vi "DropletDB-GFV.vi"(8 "error in (no error)":errorcluster, 10 "Data in":variant, 11 "Command In":T1=enum."Init") -> (0 "error out":errorcluster, 2 "Data out":variant)   [LabVIEW 2013]
uses:
  DbEnum.ctl
  TypeDef/GreyLevelData.ctl
  TypeDef/FreezePointData.ctl
  DropletDB.ctl
  ConfEnum.ctl
  ConfDB.ctl
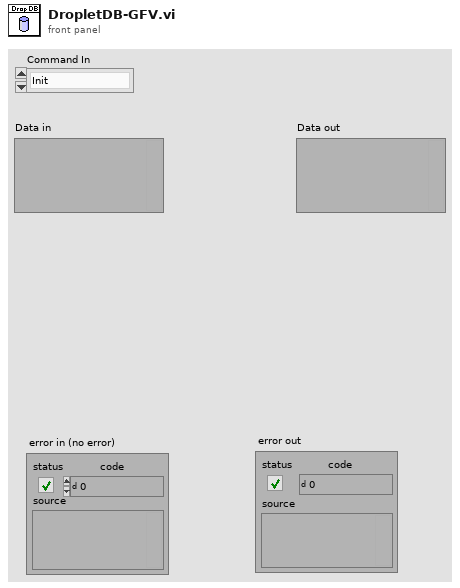
[diagram p1: front panel]
types:
  T1 = typedef "DbEnum.ctl" = enum16{"Write DropletDB", "Init", "Insert Detection Result Data", "Insert Grey Level Result", "Insert Baseline Results", "AddFreezeImagesAtCertainDroplet", "UpdateIncludeDroplet", "Insert Freeze Analysis Results", "GetDropDB", "GetNoFreezedDroplets", "GetGreyLevelAndDiff", "GetGreyLevelatIndexTime", "GetDropletsBoundingBox"}
  T2 = cluster{"Position":cluster{"x":sgl, "y":sgl}, "Angle":sgl, "Scale":sgl, "Score":sgl, "Bounding Box":cluster{"x":sgl, "y":sgl}[]}[]
  T3 = typedef "DropletDB.ctl" = cluster{"ImageFreezeIndex":i32, "DropIndex":i32, "Position":cluster{"x":sgl, "y":sgl}, "Bounding Box":cluster{"x":sgl, "y":sgl}[], "Score":sgl, "GreyLevelInBoundingBox":dbl[], "GLDifference":dbl[], "Baseline level":dbl, "Peak":cluster{"Value":dbl, "Index":u32}, "Peak Onset":cluster{"Value":dbl, "Index":u32}, "FreezeFileName":string, "FreezeAbsTime":timestamp, "FreezeTemperature":dbl, "ImageIndexArray":u32[], "Freeze Point Found":bool, "Baseline std":dbl, "FreezedImageArray":cluster{"Image":u8[][]}[], "Include Droplet":bool, "Remark":string, "Freeze Rel Time":u32[]}[]
  T4 = typedef "GreyLevelData.ctl" = cluster{"Grey Level":dbl[], "Grey level diff":dbl[], "ImageIndex":u32, "Drop Index":u32}
  T5 = typedef "FreezePointData.ctl" = cluster{"Freeze YesNo":cluster{"Freeze Grey Diff value":dbl, "Freeze Point Found":bool, "Freeze Indices":u32[]}[], "Rel Time":u32[]}
  T6 = cluster{"DropletBaseline":dbl[], "DropletBaselineSTD":dbl[]}
  T7 = typedef "ConfDB.ctl" = cluster{"NumberOfImages":i32, "NoImages2SaveAroundFreeze":i32, "Path":path, "NameOfPartialFile":string, "StartIndex":i32, "NumberOfStdTol":i32, "Detla t (sec)":i32, "Number of images for baseline":i32, "Temperature File Name":string, "Score":dbl, "Index number of Files":i32[], "End Index":i32, "Temperature Array":dbl[], "TStartIndex":i32}
  T8 = typedef "ConfEnum.ctl" = enum16{"Init", "GetConfDB", "GetTemperatureAtIndex", "WriteConfDB", "Configure DB"}
  T9 = cluster{"ImageFreezeIndex":i32, "DropIndex":i32, "Position":cluster{"x":sgl, "y":sgl}, "Bounding Box":cluster{"x":sgl, "y":sgl}[], "Score":sgl, "GreyLevelInBoundingBox":dbl[], "GLDifference":dbl[], "Baseline level":dbl, "Peak":cluster{"Value":dbl, "Index":u32}, "Peak Onset":cluster{"Value":dbl, "Index":u32}, "FreezeFileName":string, "FreezeAbsTime":timestamp, "FreezeTemperature":dbl, "ImageIndexArray":u32[], "Freeze Point Found":bool, "Baseline std":dbl, "FreezedImageArray":cluster{"Image":u8[][]}[], "Include Droplet":bool, "Remark":string, "Freeze Rel Time":u32[]}
  T10 = cluster{"Freeze Grey Diff value":dbl, "Freeze Point Found":bool, "Freeze Indices":u32[]}[]
  T11 = cluster{"ImageFreezeIndex":i32, "DropIndex":i32, "Position":cluster{"x":sgl, "y":sgl}, "Bounding Box":cluster{"x":sgl, "y":sgl}[], "Score":sgl, "GreyLevelInBoundingBox":dbl[], "GLDifference":dbl[], "Baseline level":dbl, "Peak":cluster{"Value":dbl, "Index":u32}, "Peak Onset":cluster{"Value":dbl, "Index":u32}, "FreezeFileName":string, "FreezeAbsTime":timestamp, "FreezeTemperature":dbl, "ImageIndexArray":u32[], "Freeze Point Found":bool, "Baseline std":dbl, "FreezedImageArray":cluster{"Image":u8[][]}[], "Include Droplet":bool, "Remark":string, "Freeze Rel Time":u32[]}[]
  T12 = cluster{"ImageIndexArray":u32[], "GreyLevelInBoundingBox":dbl[][], "GLDifference":dbl[][]}
  T13 = typedef "Image Type" = u32
  T14 = typedef "IMAQ Image.ctl" = refnum<image>
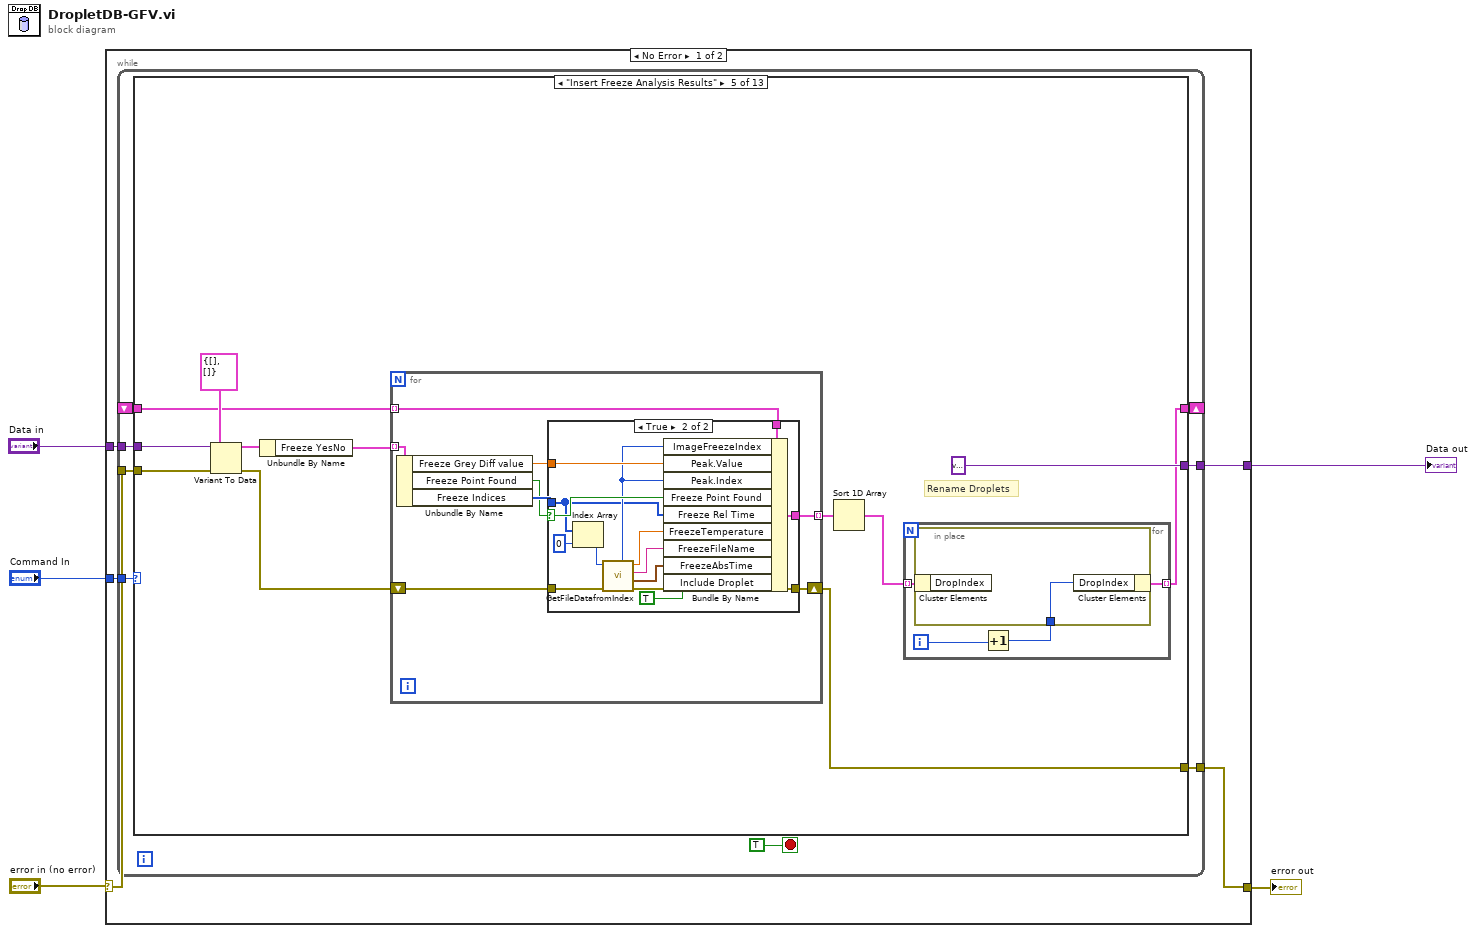
[diagram p0: block diagram]
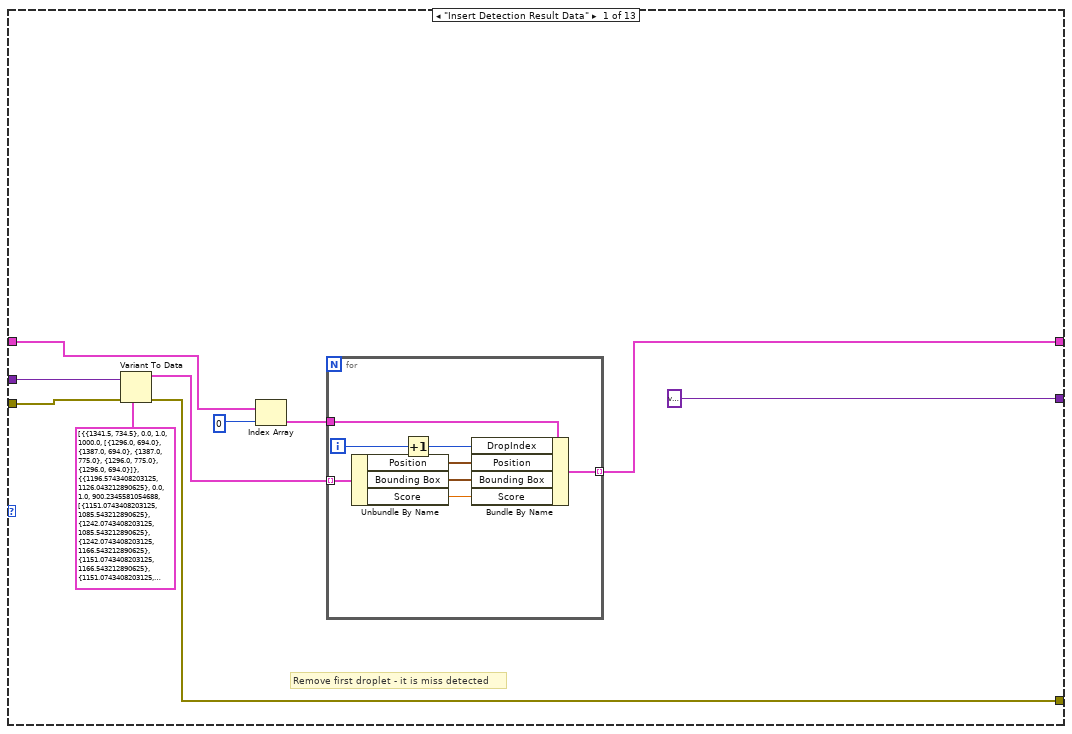
[diagram p2: hidden frame]
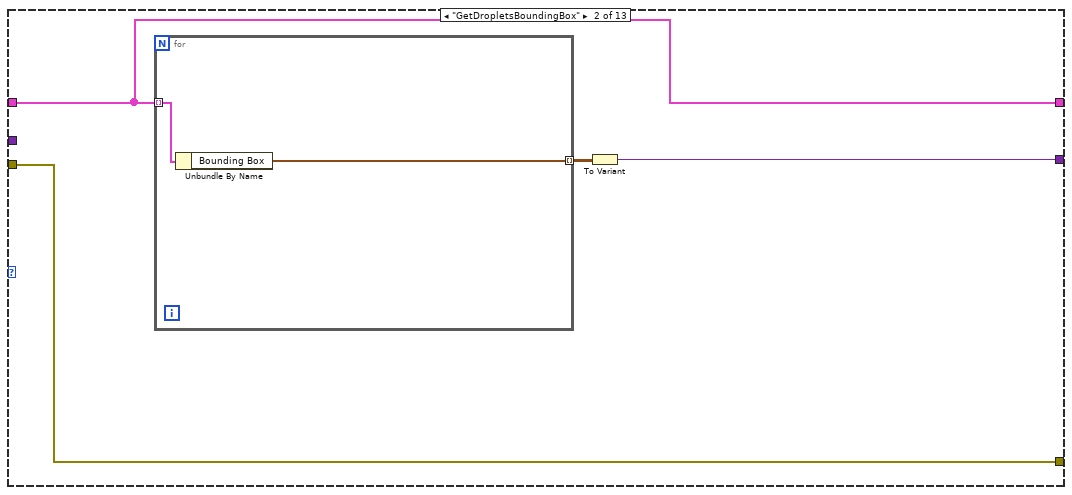
[diagram p3: hidden frame]
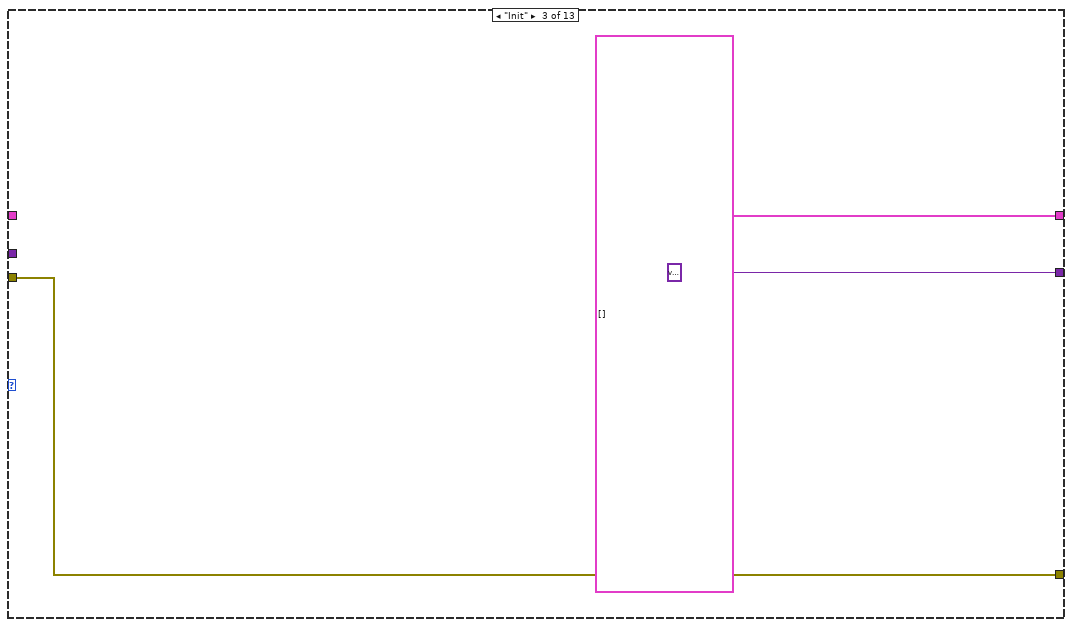
[diagram p4: hidden frame]
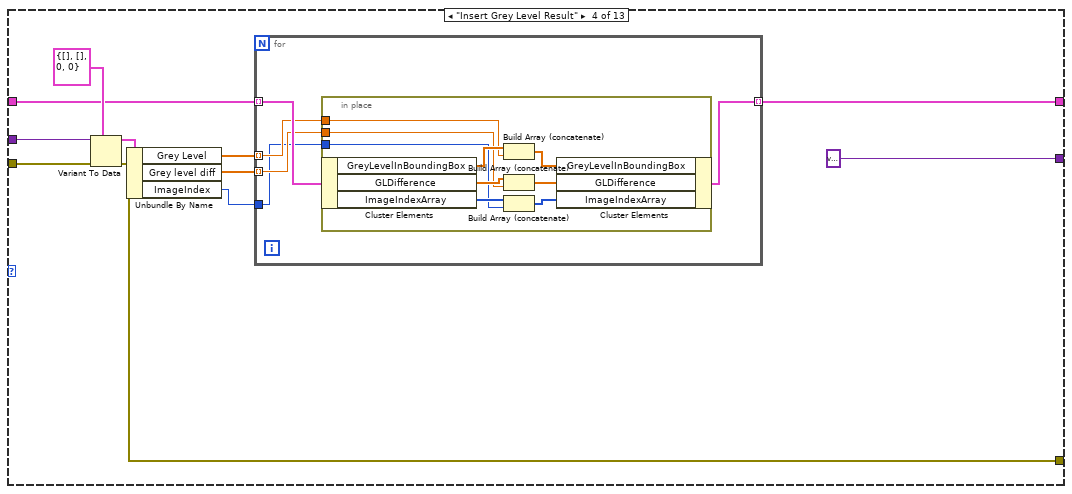
[diagram p5: hidden frame]
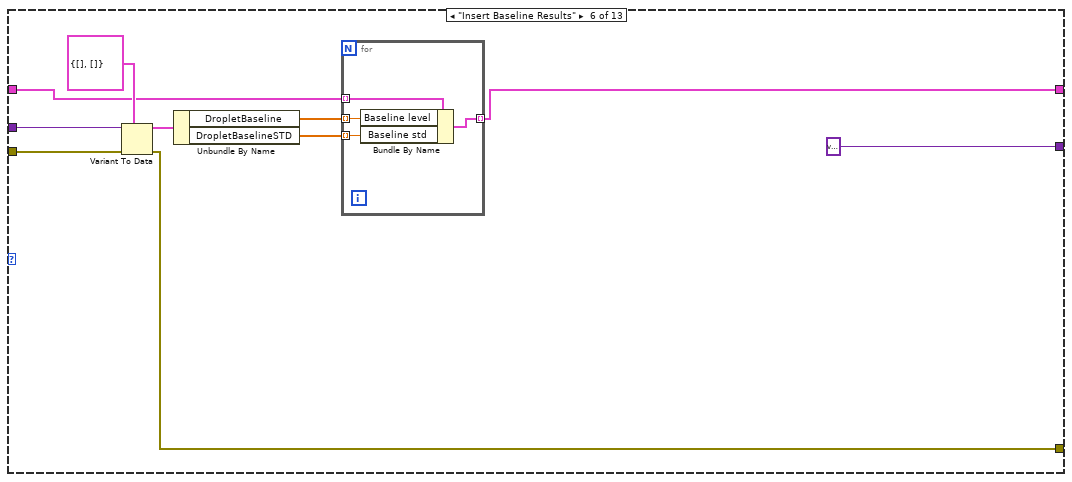
[diagram p7: hidden frame]
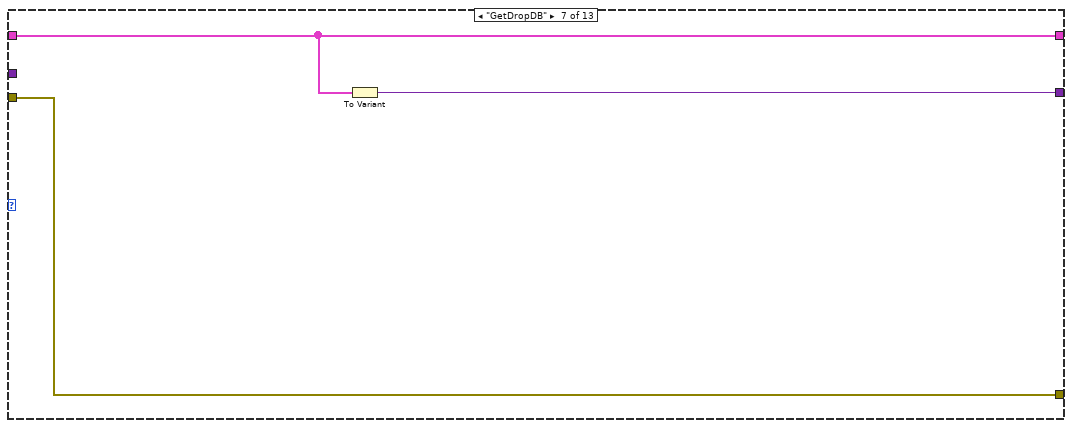
[diagram p8: hidden frame]
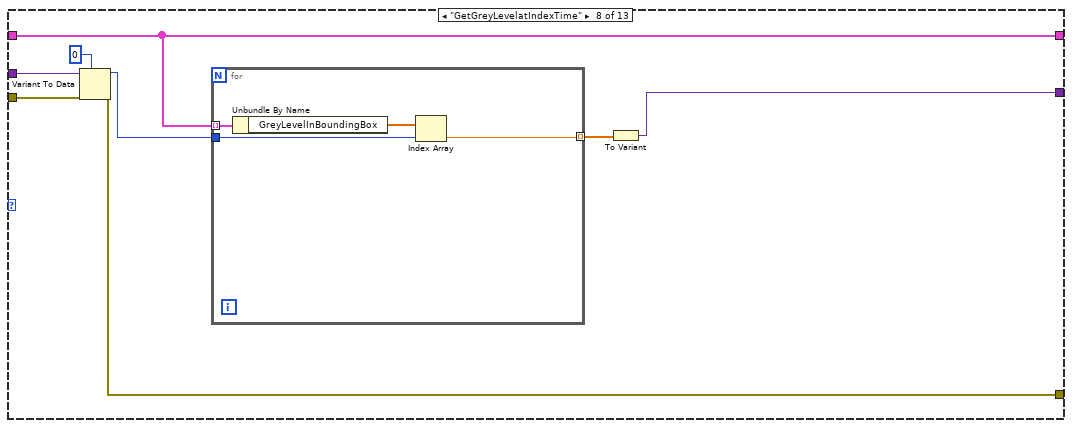
[diagram p9: hidden frame]
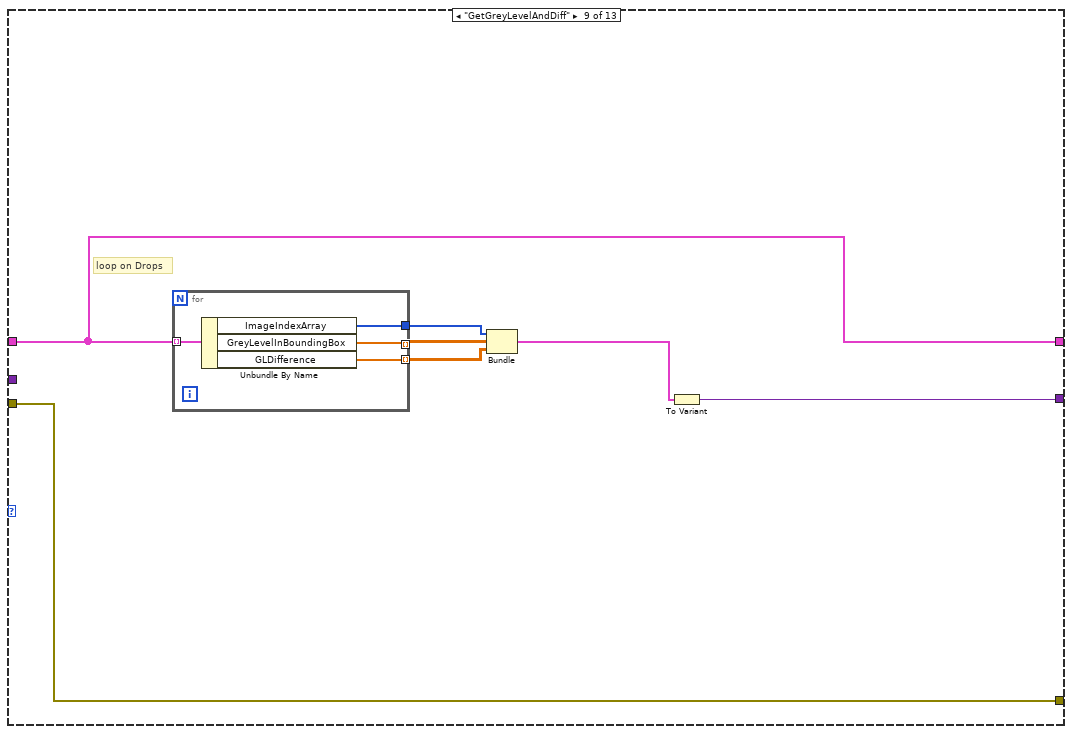
[diagram p10: hidden frame]
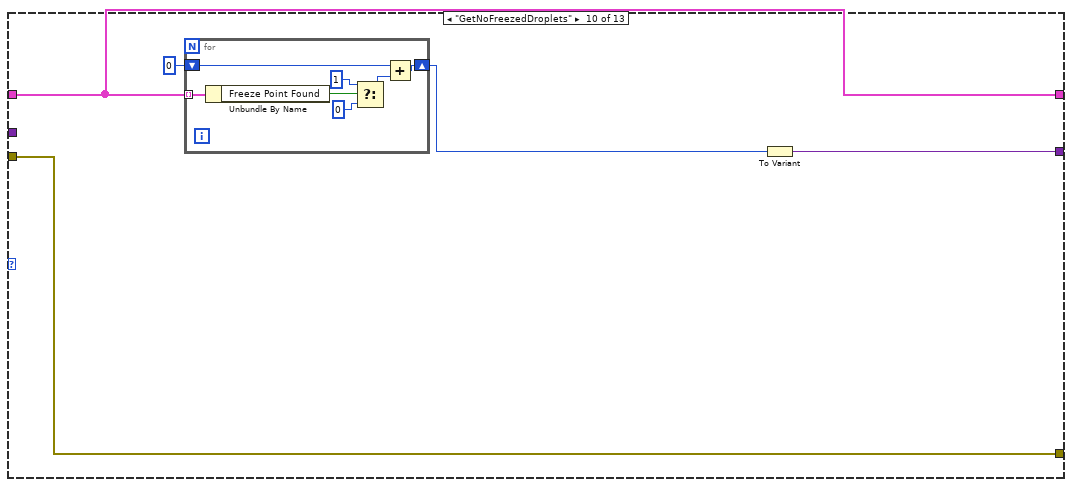
[diagram p11: hidden frame]
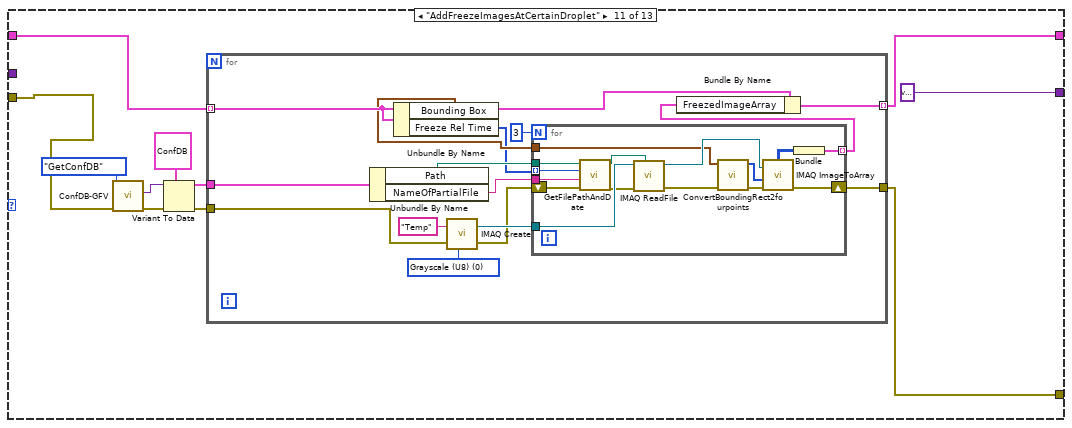
[diagram p12: hidden frame]
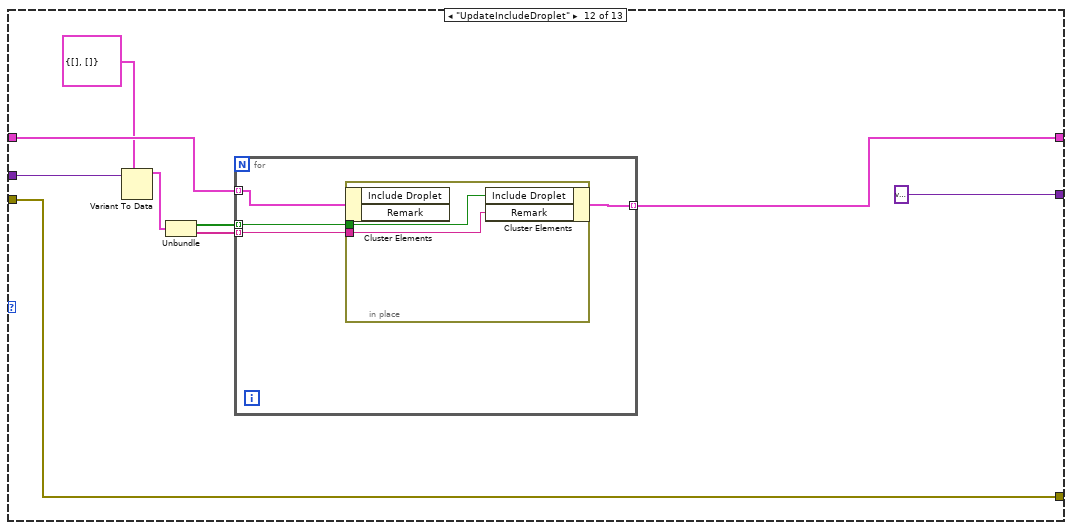
[diagram p13: hidden frame]
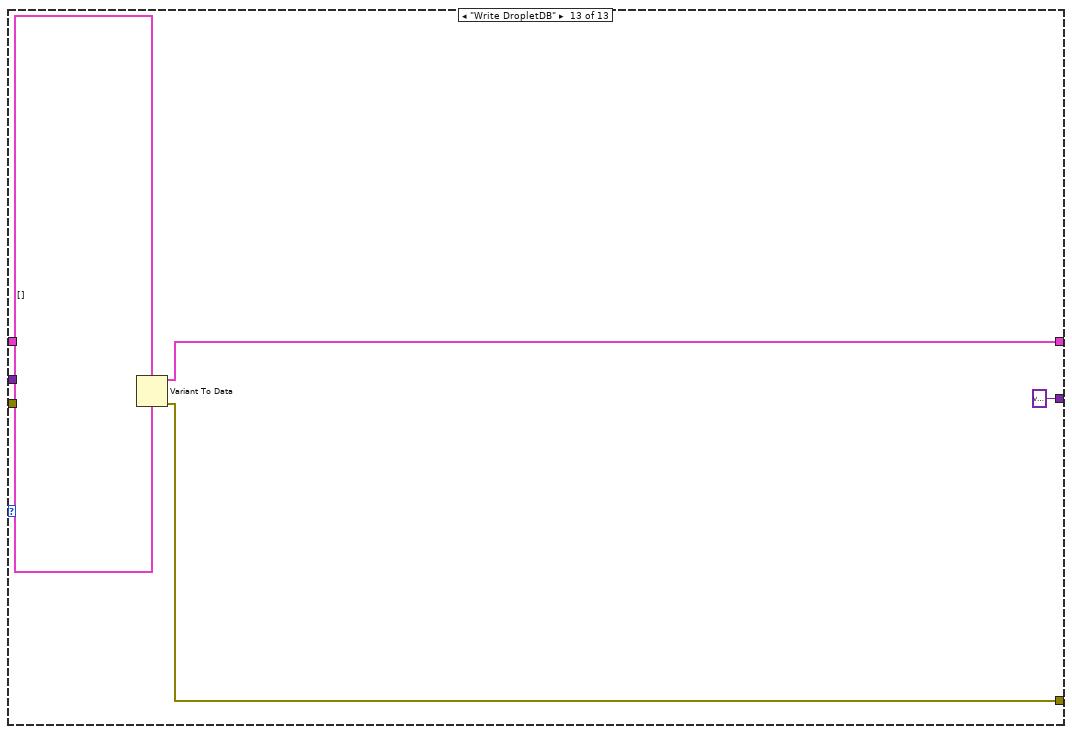
[diagram p14: hidden frame]
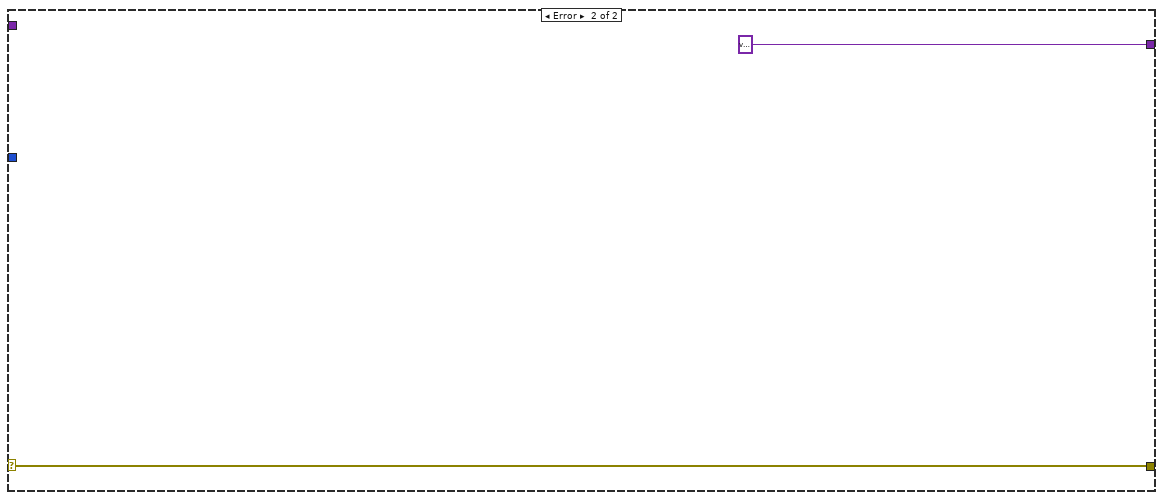
[diagram p15: hidden frame]
diagram:
  n1 = case shown="No Error" "error in (no error)" {
    selector: "error in (no error)" -> [w7 w227]
    tunnel: [w6 w227] -> w4
    tunnel: "Command In" -> [w10 _]
    tunnel: "Data in" -> [w9 _]
    tunnel: [w8 variant ("Variant")] -> w1
    frame No Error {
      n2 = while {
        tunnel: w10 -> [w17]
        shift-right: [w16] -> _
        shift-left: _ -> [w14]
        tunnel: w9 -> [w15]
        tunnel: [w13] -> w8
        tunnel: w7 -> [w12]
        tunnel: [w11] -> w6
        stop <- TRUE stop-if-true
        n3 = case shown="\"Insert Freeze Analysis Results\"" w17 {
          tunnel: [w22 w40 T3 [] ("DropletArray") w47 w72 w114 w128 w134 w147 w155 w166 w209 w222] -> w16
          tunnel: w15 -> [w28 _ _ w56 w82 w120 _ w136 _ _ _ w211 w225]
          tunnel: w14 -> [w23 w40 _ w50 w78 w118 w128 w134 w147 w155 w165 w210 _]
          tunnel: [variant ("Variant") w38 variant ("Variant") variant ("Variant") variant ("Variant") variant ("Variant") w127 w131 w146 w154 variant ("Variant") variant ("Variant") variant ("Variant")] -> w13
          tunnel: w12 -> [w20 w37 w43 w52 w81 w121 w126 w130 w141 w152 w164 w213 w224]
          tunnel: [w19 w37 w43 w51 w75 w112 w126 w129 w141 w152 w167 w213 w221] -> w11
          frame "Insert Detection Result Data" {
            # "Remove first droplet - it is miss detected"
            n4 = Variant To Data(error in=w20, type=T2 [{"Position"={"x"=1341.5, "y"=734.5}, "Angle"=0.0, "Scale"=1.0, "Score"=1000.0, "Bounding Box"=[{"x"=1296.0, "y"=694.0}, {"x"=1387.0, "y"=694.0}, {"x"=1387.0, "y"=775.0}, {"x"=1296.0, "y"=775.0}, {"x"=1296.0, "y"=694.0}]}, {"Position"={"x"=1196.5743, "y"=1126.0432}, "Angle"=0.0, "Scale"=1.0, "Score"=900.23456, "Bounding Box"=[{"x"=1151.0743, "y"=1085.5432}, {"x"=1242.0743, "y"=1085.5432}, {"x"=1242.0743, "y"=1166.5432}, {"x"=1151.0743, "y"=1166.5432}, {"x"=1151.0743, "y"=1085.5432}]}, {"Position"={"x"=1545.7823, "y"=532.04376}, "Angle"=0.0, "Scale"=1.0, "Score"=892.0734, "Bounding Box"=[{"x"=1500.2823, "y"=491.54376}, {"x"=1591.2823, "y"=491.54376}, {"x"=1591.2823, "y"=572.54376}, {"x"=1500.2823, "y"=572.54376}, {"x"=1500.2823, "y"=491.54376}]}, {"Position"={"x"=1094.883, "y"=753.2342}, "Angle"=0.0, "Scale"=1.0, "Score"=891.1741, "Bounding Box"=[{"x"=1049.383, "y"=712.7342}, {"x"=1140.383, "y"=712.7342}, {"x"=1140.383, "y"=793.7342}, {"x"=1049.383, "y"=793.7342}, {"x"=1049.383, "y"=712.7342}]}, {"Position"={"x"=1371.3896, "y"=961.625}, "Angle"=0.0, "Scale"=1.0, "Score"=878.96686, "Bounding Box"=[{"x"=1325.8896, "y"=921.125}, {"x"=1416.8896, "y"=921.125}, {"x"=1416.8896, "y"=1002.125}, {"x"=1325.8896, "y"=1002.125}, {"x"=1325.8896, "y"=921.125}]}, {"Position"={"x"=1686.145, "y"=812.43805}, "Angle"=0.0, "Scale"=1.0, "Score"=825.67773, "Bounding Box"=[{"x"=1640.645, "y"=771.93805}, {"x"=1731.645, "y"=771.93805}, {"x"=1731.645, "y"=852.93805}, {"x"=1640.645, "y"=852.93805}, {"x"=1640.645, "y"=771.93805}]}, {"Position"={"x"=936.9166, "y"=624.4227}, "Angle"=0.0, "Scale"=1.0, "Score"=817.7966, "Bounding Box"=[{"x"=891.4166, "y"=583.9227}, {"x"=982.4166, "y"=583.9227}, {"x"=982.4166, "y"=664.9227}, {"x"=891.4166, "y"=664.9227}, {"x"=891.4166, "y"=583.9227}]}, {"Position"={"x"=1536.802, "y"=1190.3126}, "Angle"=0.0, "Scale"=1.0, "Score"=786.6126, "Bounding Box"=[{"x"=1491.302, "y"=1149.8126}, {"x"=1582.302, "y"=1149.8126}, {"x"=1582.302, "y"=1230.8126}, {"x"=1491.302, "y"=1230.8126}, {"x"=1491.302, "y"=1149.8126}]}, {"Position"={"x"=1679.4249, "y"=1001.6944}, "Angle"=0.0, "Scale"=1.0, "Score"=784.3884, "Bounding Box"=[{"x"=1633.9249, "y"=961.1944}, {"x"=1724.9249, "y"=961.1944}, {"x"=1724.9249, "y"=1042.1943}, {"x"=1633.9249, "y"=1042.1943}, {"x"=1633.9249, "y"=961.1944}]}, {"Position"={"x"=1229.3533, "y"=500.3024}, "Angle"=0.0, "Scale"=1.0, "Score"=773.35645, "Bounding Box"=[{"x"=1183.8533, "y"=459.8024}, {"x"=1274.8533, "y"=459.8024}, {"x"=1274.8533, "y"=540.80237}, {"x"=1183.8533, "y"=540.80237}, {"x"=1183.8533, "y"=459.8024}]}, {"Position"={"x"=951.5936, "y"=1321.2926}, "Angle"=0.0, "Scale"=1.0, "Score"=751.618, "Bounding Box"=[{"x"=906.0936, "y"=1280.7926}, {"x"=997.0936, "y"=1280.7926}, {"x"=997.0936, "y"=1361.7926}, {"x"=906.0936, "y"=1361.7926}, {"x"=906.0936, "y"=1280.7926}]}, {"Position"={"x"=1773.0933, "y"=552.07654}, "Angle"=0.0, "Scale"=1.0, "Score"=723.29376, "Bounding Box"=[{"x"=1727.5933, "y"=511.57654}, {"x"=1818.5933, "y"=511.57654}, {"x"=1818.5933, "y"=592.57654}, {"x"=1727.5933, "y"=592.57654}, {"x"=1727.5933, "y"=511.57654}]}, {"Position"={"x"=1248.5851, "y"=325.4367}, "Angle"=0.0, "Scale"=1.0, "Score"=719.0533, "Bounding Box"=[{"x"=1203.0851, "y"=284.9367}, {"x"=1294.0851, "y"=284.9367}, {"x"=1294.0851, "y"=365.9367}, {"x"=1203.0851, "y"=365.9367}, {"x"=1203.0851, "y"=284.9367}]}, {"Position"={"x"=1253.8042, "y"=1431.3312}, "Angle"=0.0, "Scale"=1.0, "Score"=717.0521, "Bounding Box"=[{"x"=1208.3042, "y"=1390.8312}, {"x"=1299.3042, "y"=1390.8312}, {"x"=1299.3042, "y"=1471.8312}, {"x"=1208.3042, "y"=1471.8312}, {"x"=1208.3042, "y"=1390.8312}]}, {"Position"={"x"=1508.0845, "y"=1397.7313}, "Angle"=0.0, "Scale"=1.0, "Score"=702.3233, "Bounding Box"=[{"x"=1462.5845, "y"=1357.2313}, {"x"=1553.5845, "y"=1357.2313}, {"x"=1553.5845, "y"=1438.2313}, {"x"=1462.5845, "y"=1438.2313}, {"x"=1462.5845, "y"=1357.2313}]}, {"Position"={"x"=1552.1433, "y"=304.62778}, "Angle"=0.0, "Scale"=1.0, "Score"=694.1083, "Bounding Box"=[{"x"=1506.6433, "y"=264.12778}, {"x"=1597.6433, "y"=264.12778}, {"x"=1597.6433, "y"=345.12778}, {"x"=1506.6433, "y"=345.12778}, {"x"=1506.6433, "y"=264.12778}]}, {"Position"={"x"=786.0882, "y"=1109.9098}, "Angle"=0.0, "Scale"=1.0, "Score"=691.0762, "Bounding Box"=[{"x"=740.5882, "y"=1069.4098}, {"x"=831.5882, "y"=1069.4098}, {"x"=831.5882, "y"=1150.4098}, {"x"=740.5882, "y"=1150.4098}, {"x"=740.5882, "y"=1069.4098}]}, {"Position"={"x"=1926.0133, "y"=864.04224}, "Angle"=0.0, "Scale"=1.0, "Score"=639.03375, "Bounding Box"=[{"x"=1880.5133, "y"=823.54224}, {"x"=1971.5133, "y"=823.54224}, {"x"=1971.5133, "y"=904.54224}, {"x"=1880.5133, "y"=904.54224}, {"x"=1880.5133, "y"=823.54224}]}, {"Position"={"x"=1927.5698, "y"=665.46716}, "Angle"=0.0, "Scale"=1.0, "Score"=624.3622, "Bounding Box"=[{"x"=1882.0698, "y"=624.96716}, {"x"=1973.0698, "y"=624.96716}, {"x"=1973.0698, "y"=705.96716}, {"x"=1882.0698, "y"=705.96716}, {"x"=1882.0698, "y"=624.96716}]}, {"Position"={"x"=1036.6719, "y"=924.2498}, "Angle"=0.0, "Scale"=1.0, "Score"=622.71356, "Bounding Box"=[{"x"=991.1719, "y"=883.7498}, {"x"=1082.1719, "y"=883.7498}, {"x"=1082.1719, "y"=964.7498}, {"x"=991.1719, "y"=964.7498}, {"x"=991.1719, "y"=883.7498}]}, {"Position"={"x"=1798.4291, "y"=427.18503}, "Angle"=0.0, "Scale"=1.0, "Score"=612.04645, "Bounding Box"=[{"x"=1752.9291, "y"=386.68503}, {"x"=1843.9291, "y"=386.68503}, {"x"=1843.9291, "y"=467.68503}, {"x"=1752.9291, "y"=467.68503}, {"x"=1752.9291, "y"=386.68503}]}, {"Position"={"x"=679.48035, "y"=781.2287}, "Angle"=0.0, "Scale"=1.0, "Score"=604.38666, "Bounding Box"=[{"x"=633.98035, "y"=740.7287}, {"x"=724.98035, "y"=740.7287}, {"x"=724.98035, "y"=821.7287}, {"x"=633.98035, "y"=821.7287}, {"x"=633.98035, "y"=740.7287}]}, {"Position"={"x"=1858.5896, "y"=1175.5317}, "Angle"=0.0, "Scale"=1.0, "Score"=601.6367, "Bounding Box"=[{"x"=1813.0896, "y"=1135.0317}, {"x"=1904.0896, "y"=1135.0317}, {"x"=1904.0896, "y"=1216.0317}, {"x"=1813.0896, "y"=1216.0317}, {"x"=1813.0896, "y"=1135.0317}]}, {"Position"={"x"=873.6445, "y"=427.1809}, "Angle"=0.0, "Scale"=1.0, "Score"=584.28125, "Bounding Box"=[{"x"=828.1445, "y"=386.6809}, {"x"=919.1445, "y"=386.6809}, {"x"=919.1445, "y"=467.6809}, {"x"=828.1445, "y"=467.6809}, {"x"=828.1445, "y"=386.6809}]}, {"Position"={"x"=599.6848, "y"=551.81195}, "Angle"=0.0, "Scale"=1.0, "Score"=543.92706, "Bounding Box"=[{"x"=554.1848, "y"=511.31195}, {"x"=645.1848, "y"=511.31195}, {"x"=645.1848, "y"=592.31195}, {"x"=554.1848, "y"=592.31195}, {"x"=554.1848, "y"=511.31195}]}] ("Matches (pixel)"), Variant=w28) -> (data=w24:T2, error out=w19:errorcluster)
            n5 = Index Array(array=w23, index=0) -> (element=w25:T9)
            n6 = for {
              tunnel: w24 -> [w31] mode=indexing
              tunnel: [w33] -> w22 mode=indexing
              tunnel: w25 -> [w32]
              i -> [w30]
              n7 = Unbundle By Name(w31) -> ("Position"=w36:cluster{"x":sgl, "y":sgl}, "Bounding Box"=w35:cluster{"x":sgl, "y":sgl}[], "Score"=w34:sgl)
              n8 = Increment(x=w30) -> (x+1=w29:i32)
              n9 = Bundle By Name(cluster=w32, "DropIndex"=w29, "Position"=w36, "Bounding Box"=w35, "Score"=w34) -> (w33:T9)
            }
          }
          frame "GetDropletsBoundingBox" {
            n10 = for {
              tunnel: w40 -> [w42] mode=indexing
              tunnel: [w41] -> w39 mode=indexing
              n11 = Unbundle By Name(w42) -> ("Bounding Box"=w41:cluster{"x":sgl, "y":sgl}[])
            }
            n12 = To Variant(anything=w39) -> (Variant=w38:variant)
          }
          frame "Init" {
          }
          frame "Insert Grey Level Result" {
            n13 = Variant To Data(error in=w52, type=T4 {"Grey Level"=[], "Grey level diff"=[], "ImageIndex"=0, "Drop Index"=0} ("Cluster"), Variant=w56) -> (data=w54:T4, error out=w51:errorcluster)
            n14 = Unbundle By Name(w54) -> ("Grey Level"=w49:dbl[], "Grey level diff"=w48:dbl[], "ImageIndex"=w46:u32)
            n15 = for {
              tunnel: w50 -> [w61] mode=indexing
              tunnel: w49 -> [w60] mode=indexing
              tunnel: w48 -> [w59] mode=indexing
              tunnel: [w58] -> w47 mode=indexing
              tunnel: w46 -> [w57]
              n16 = in-place {
                in-place-border: w60 -> [w68]
                in-place-border: w59 -> [w65]
                in-place-border: w57 -> [w62]
                n17 = in-place-cluster #1(w61) -> ("GreyLevelInBoundingBox"=w70:dbl[], "GLDifference"=w67:dbl[], "ImageIndexArray"=w64:u32[])
                n18 = Build Array (concatenate)(w70, w68) -> (w69:dbl[])
                n19 = Build Array (concatenate)(w67, w65) -> (w66:dbl[])
                n20 = Build Array (concatenate)(w64, w62) -> (w63:u32[])
                n21 = in-place-cluster #1("GreyLevelInBoundingBox"=w69, "GLDifference"=w66, "ImageIndexArray"=w63) -> (w58:T9)
              }
            }
          }
          frame "Insert Freeze Analysis Results" {
            # "Rename Droplets"
            n22 = Variant To Data(error in=w81, type=T5 {"Freeze YesNo"=[], "Rel Time"=[]} ("Freeze YesNo"), Variant=w82) -> (data=w77:T5, error out=w71:errorcluster)
            n23 = Unbundle By Name(w77) -> ("Freeze YesNo"=w76:T10)
            n24 = for {
              tunnel: w76 -> [w95] mode=indexing
              tunnel: w78 -> [w94] mode=indexing
              tunnel: [w92] -> w74 mode=indexing
              shift-right: [w90] -> w75
              shift-left: w71 -> [w91]
              n25 = Unbundle By Name(w95) -> ("Freeze Grey Diff value"=w93:dbl, "Freeze Point Found"=w88:bool, "Freeze Indices"=w89:u32[])
              n26 = case shown="True" w88 {
                selector: w88 -> [_ w103]
                tunnel: w94 -> [w97 w111]
                tunnel: w93 -> [_ w110]
                tunnel: [w97 w109] -> w92
                tunnel: w91 -> [w96 w108]
                tunnel: [w96 w107] -> w90
                tunnel: w89 -> [_ w100]
                frame False {
                }
                frame True {
                  n27 = Index Array(array=w100, index=0) -> (element=w98:u32)
                  n28 = call "GetFileDatafromIndex.vi"("Error In"=w108, "DuplicateFilteredIndex"=w98) -> ("Error Out"=w107:errorcluster, "FreezeAbsTime"=w104:timestamp, "FreezeFileName"=w105:string, "FreezeTemperature"=w106:dbl, "Peak index"=w102:u32)  [unwired: 5 in]
                  n29 = Bundle By Name(cluster=w111, "ImageFreezeIndex"=w102, "Peak.Value"=w110, "Peak.Index"=w102, "Freeze Point Found"=w103, "Freeze Rel Time"=w100, "FreezeTemperature"=w106, "FreezeFileName"=w105, "FreezeAbsTime"=w104, "Include Droplet"=TRUE) -> (w109:T9)
                }
              }
            }
            n30 = Sort 1D Array(array=w74) -> (sorted array=w73:T11)
            n31 = for {
              tunnel: w73 -> [w86] mode=indexing
              tunnel: [w85] -> w72 mode=indexing
              i -> [w84]
              n32 = Increment(x=w84) -> (x+1=w83:i32)
              n33 = in-place {
                in-place-border: w83 -> [w87]
                n34 = in-place-cluster #2(w86) -> ()  [unwired: 1 out]
                n35 = in-place-cluster #2("DropIndex"=w87) -> (w85:T9)
              }
            }
          }
          frame "Insert Baseline Results" {
            n36 = Variant To Data(error in=w121, type=T6 {"DropletBaseline"=[], "DropletBaselineSTD"=[]} ("output cluster"), Variant=w120) -> (data=w117:T6, error out=w112:errorcluster)
            n37 = Unbundle By Name(w117) -> ("DropletBaseline"=w116:dbl[], "DropletBaselineSTD"=w115:dbl[])
            n38 = for {
              tunnel: w118 -> [w125] mode=indexing
              tunnel: w116 -> [w124] mode=indexing
              tunnel: w115 -> [w122] mode=indexing
              tunnel: [w123] -> w114 mode=indexing
              n39 = Bundle By Name(cluster=w125, "Baseline level"=w124, "Baseline std"=w122) -> (w123:T9)
            }
          }
          frame "GetDropDB" {
            n40 = To Variant(anything=w128) -> (Variant=w127:variant)
          }
          frame "GetGreyLevelatIndexTime" {
            n41 = Variant To Data(error in=w130, type=0 ("x-y"), Variant=w136) -> (data=w133:i32, error out=w129:errorcluster)
            n42 = for {
              tunnel: w134 -> [w140] mode=indexing
              tunnel: w133 -> [w138]
              tunnel: [w137] -> w132 mode=indexing
              n43 = Unbundle By Name(w140) -> ("GreyLevelInBoundingBox"=w139:dbl[])
              n44 = Index Array(array=w139, index=w138) -> (element=w137:dbl)
            }
            n45 = To Variant(anything=w132) -> (Variant=w131:variant)
          }
          frame "GetGreyLevelAndDiff" {
            # "loop on Drops"
            n46 = for {
              tunnel: w147 -> [w151] mode=indexing
              tunnel: [w150] -> w144 mode=indexing
              tunnel: [w149] -> w143 mode=indexing
              tunnel: [w148] -> w145
              n47 = Unbundle By Name(w151) -> ("ImageIndexArray"=w148:u32[], "GreyLevelInBoundingBox"=w150:dbl[], "GLDifference"=w149:dbl[])
            }
            n48 = Bundle("ImageIndexArray"=w145, "GreyLevelInBoundingBox"=w144, "GLDifference"=w143) -> (w142:T12)  [unwired: 1 in]
            n49 = To Variant(anything=w142) -> (Variant=w146:variant)
          }
          frame "GetNoFreezedDroplets" {
            n50 = for {
              tunnel: w155 -> [w163] mode=indexing
              shift-right: [w158] -> w153
              shift-left: u32 0 -> [w157]
              n51 = Unbundle By Name(w163) -> ("Freeze Point Found"=w162:bool)
              n52 = Select(t=u32 1, s=w162, f=u32 0) -> (s? t:f=w161:u32)
              n53 = Add(x=w157, y=w161) -> (x+y=w158:u32)
            }
            n54 = To Variant(anything=w153) -> (Variant=w154:variant)
          }
          frame "AddFreezeImagesAtCertainDroplet" {
            n55 = call "ConfDB-GFV.vi"("error in (no error)"=w164, "Command In"=ConfEnum."GetConfDB") -> ("error out"=w171:errorcluster, "Data out"=w172:variant)  [unwired: 8 in]
            n56 = Variant To Data(error in=w171, type=T7 {"NumberOfImages"=0, "NoImages2SaveAroundFreeze"=0, "Path"=path "", "NameOfPartialFile"="", "StartIndex"=0, "NumberOfStdTol"=0, "Detla t (sec)"=0, "Number of images for baseline"=0, "Temperature File Name"="", "Score"=0.0, "Index number of Files"=[], "End Index"=0, "Temperature Array"=[], "TStartIndex"=0} ("ConfDB"), Variant=w172) -> (data=w169:T7, error out=w168:errorcluster)
            n57 = for {
              tunnel: w169 -> [w189]
              tunnel: w168 -> [w188]
              tunnel: [w187] -> w167
              tunnel: w165 -> [w185] mode=indexing
              tunnel: [w186] -> w166 mode=indexing
              w182 = T13 0 items=["Grayscale (U8)", "Grayscale (I16)", "Grayscale (SGL)", "Complex (CSG)", "RGB (U32)", "HSL (U32)", "RGB (U64)", "Grayscale (U16)"] ("Image Type")
              n58 = Unbundle By Name(w189) -> ("Path"=w184:path, "NameOfPartialFile"=w183:string)
              n59 = Unbundle By Name(w185) -> ("Bounding Box"=w176:cluster{"x":sgl, "y":sgl}[], "Freeze Rel Time"=w175:u32[])
              n60 = call "IMAQ Create"("Image Name"="Temp", "Image Type"=w182, "error in (no error)"=w188) -> ("New Image"=w180:T14, "error out"=w179:errorcluster)  [unwired: 1 in, 1 out]
              n61 = for {
                N: 3 -> [_]
                tunnel: w184 -> [w204]
                tunnel: w183 -> [w203]
                tunnel: w180 -> [w201]
                tunnel: [w193] -> w177 mode=indexing
                shift-right: [w192] -> w187
                shift-left: w179 -> [w195]
                tunnel: w176 -> [w191]
                tunnel: w175 -> [w190] mode=indexing
                n62 = call "GetFilePathAndDate.vi"("error in (no error)"=w195, "String"=w203, "Index"=w190, "Path"=w204) -> ("error out"=w196:errorcluster, "file out"=w202:path)  [unwired: 5 in, 1 out]
                n63 = call "IMAQ ReadFile"("File Path"=w202, "error in (no error)"=w196, "Image"=w201) -> ("error out"=w197:errorcluster, "Image Out"=w198:T14)  [unwired: 2 in, 5 out]
                n64 = call "ConvertBoundingRect2fourpoints.vi"("Error In"=w197, "Bounding Box"=w191) -> ("Error Out"=w200:errorcluster, "Array"=w199:i32[])  [unwired: 8 in]
                n65 = call "IMAQ ImageToArray"("error in (no error)"=w200, "Optional Rectangle"=w199, "Image"=w198) -> ("error out"=w192:errorcluster, "Image Pixels (U8)"=w194:u8[][])  [unwired: 1 in, 3 out]
                n66 = Bundle("Image Pixels (U8)"=w194) -> (w193:cluster{"Image Pixels (U8)":u8[][]})  [unwired: 1 in]
              }
              n67 = Bundle By Name(cluster=w185, "FreezedImageArray"=w177) -> (w186:T9)
            }
          }
          frame "UpdateIncludeDroplet" {
            n68 = Variant To Data(type=cluster{bool[], string[]} {[], []} ("cluster"), Variant=w211) -> (data=w207:cluster{bool[], string[]})  [unwired: 1 in, 1 out]
            n69 = Unbundle(w207) -> (w206:bool[], w205:string[])
            n70 = for {
              tunnel: w210 -> [w217] mode=indexing
              tunnel: [w216] -> w209 mode=indexing
              tunnel: w206 -> [w215] mode=indexing
              tunnel: w205 -> [w214] mode=indexing
              n71 = in-place {
                in-place-border: w215 -> [w219]
                in-place-border: w214 -> [w218]
                n72 = in-place-cluster #3(w217) -> ()  [unwired: 2 out]
                n73 = in-place-cluster #3("Include Droplet"=w219, "Remark"=w218) -> (w216:T9)
              }
            }
          }
          frame "Write DropletDB" {
            n74 = Variant To Data(error in=w224, type=T3 [] ("DropletArray"), Variant=w225) -> (data=w222:T3, error out=w221:errorcluster)
          }
        }
      }
    }
    frame Error {
    }
  }
  "error out" <- w4
  "Data out" <- w1
